vi "D4xxx Initialize.vi"(8 "error in (no error)":errorcluster, 10 "Reset (False)":bool, 11 "session in":T1) -> (0 "error out":errorcluster, 2 "idn string":string, 3 "session out":T1)   [LabVIEW 2020]
doc: "Intialize and configurate Fluke 5xxx."
uses:
  Fluke 5XXX/top_lev/F5xxx_session.ctl
  Fluke 5XXX/top_lev/F5xxx_output_mode.ctl
  Datron D4xxx.lvlib
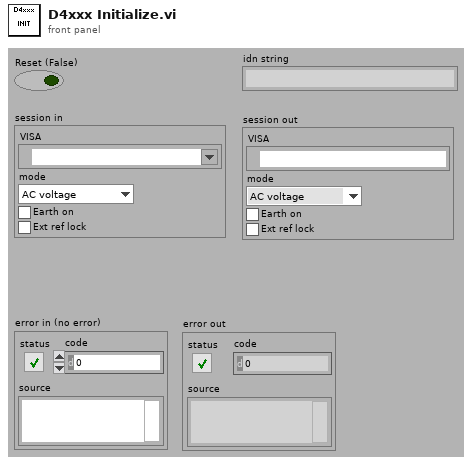
[diagram p1: front panel]
types:
  T1 = typedef "F5xxx_session.ctl" = cluster{"VISA":refnum<visa-resource-name>, "mode":T2, "Earth on":bool, "Ext ref lock":bool}
  T2 = typedef "F5xxx_output_mode.ctl" = enum16{"AC voltage", "AC current"}
  T3 = enum16{"F0 - V DC", "F1 - V AC", "F2 - A DC", "F3 - A AC", "F4 - R", "F5 - V WB"}
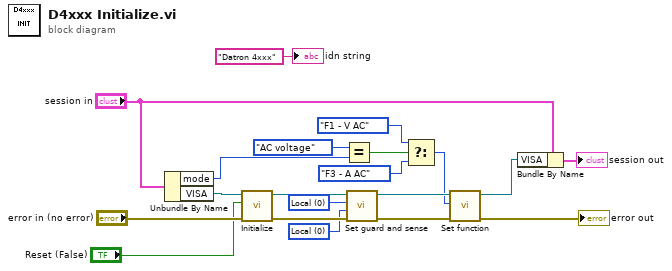
[diagram p0: block diagram]
diagram:
  w11 = u16 0 items=["Local", "Remote", "Unchanged"] ("Sense (Unchanged)")
  w12 = u16 0 items=["Local", "Remote", "Unchanged"] ("Guard (Unchanged)")
  n1 = Unbundle By Name("session in") -> ("mode"=w8:T2, "VISA"=w19:refnum<visa-resource-name>)
  n2 = call "Initialize.vi"("error in (no error)"="error in (no error)", "Reset (True)"="Reset (False)", "VISA resource name"=w19) -> ("error out"=w14:errorcluster, "VISA resource name out"=w13:refnum<visa-resource-name>)  [unwired: 7 in]
  n3 = Equal?(x=F5xxx_output_mode."AC voltage", y=w8) -> (x = y?=w6:bool)
  n4 = call "Set guard and sense.vi"("error in"=w14, "Sense (Unchanged)"=w11, "Guard (Unchanged)"=w12, "VISA resource name"=w13) -> ("error out"=w10:errorcluster, "VISA resource name out"=w9:refnum<visa-resource-name>)  [unwired: 4 in, 2 out]
  n5 = Select(t=T3."F1 - V AC" ("Function (F0 - V DC)"), s=w6, f=T3."F3 - A AC" ("Function (F0 - V DC)")) -> (s? t:f=w3:T3)
  n6 = call "Set function.vi"("error in"=w10, "Function (F0 - V DC)"=w3, "VISA resource name"=w9) -> ("error out"=→"error out":errorcluster, "VISA resource name out"=w2:refnum<visa-resource-name>)  [unwired: 7 in]
  n7 = Bundle By Name(cluster="session in", "VISA"=w2) -> (→"session out":T1)
  "idn string" <- "Datron 4xxx" ("idn string")
